vi "PH_BL-Master.PC _getVacLimits.vi"(0 "i ref in":refnum<vi>, 2 "Channelname":string="N/A", 3 "Value":dbl, 4 "no link":bool, 5 "error in (no error)":errorcluster) -> (14 "i ref out":refnum<vi>, 19 "error out":errorcluster)   [LabVIEW 2014, in "PH_BL-Master.lvlib"]
doc: "This VI writes the incoming information to own attributes."
uses:
  PH_BL-Master.lvlib
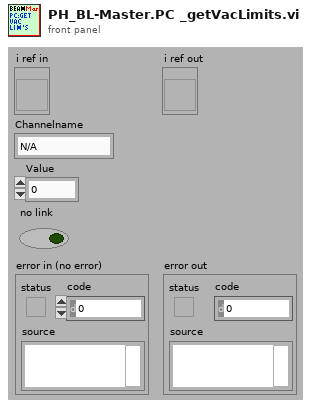
[diagram p1: front panel]
types:
  T1 = typedef "PH_BL-Master.lvlib/PH_BL-Master.i attribute.ctl" = cluster{"Remote controlled":bool, "Boolean Condition Service Subscriber":refnum<vi>[], "Picture Condition Service Subscriber":refnum<vi>[], "R2S":cluster{"GUI Ref":refnum<vi>, "State":bool}, "Vacua":cluster{"GUI Ref":refnum<vi>, "Limit":dbl, "Curr Value":dbl, "in range":bool}[], "O2 Inspection":cluster{"GUI Ref":refnum<vi>, "Concentration":dbl, "State":T2}[], "Boolean Status Service Subscriber":cluster{"GUI Ref":refnum<vi>, "Status":T2, "no Link?":bool, "Status Subscriber Class":T3}[], "Picture Status Service Subscriber":cluster{"GUI Ref":refnum<vi>, "Status":T2, "no Link?":bool, "Status Subscriber Class":T3}[], "6P 4Q Service Subscriber":cluster{"GUI Ref":refnum<vi>, "Selector":T4, "no Link?":bool}[], "Index of latest 6P 4Q changing Instance":i32, "Index of latest Picture Status changing Instance":i32, "Index of latest Boolean Status changing Instance":i32, "Vision ID on same Node":string, "Start Phase over?":bool, "GUI Ref Delete":refnum<vi>}
  T2 = typedef "PH_StatusHandler.lvlib/PH_StatusHandler.Status.ctl" = i16
  T3 = typedef "PH_BL-Master.lvlib/PH_BL-Master.Status Subscriber Class.ctl" = enum16{"unknown", "Switch", "BB", "6P Switch", "Switch GUI", "Switch and 6P State", "Force Sensor"}
  T4 = typedef "PH_4_Pos_Selector.lvlib/PH_4_Pos_Selector.Position Selector.ctl" = u16
  T5 = cluster{"GUI Ref":refnum<vi>, "Limit":dbl, "Curr Value":dbl, "in range":bool}[]
  T6 = cluster{"GUI Ref":refnum<vi>, "Limit":dbl, "Curr Value":dbl, "in range":bool}
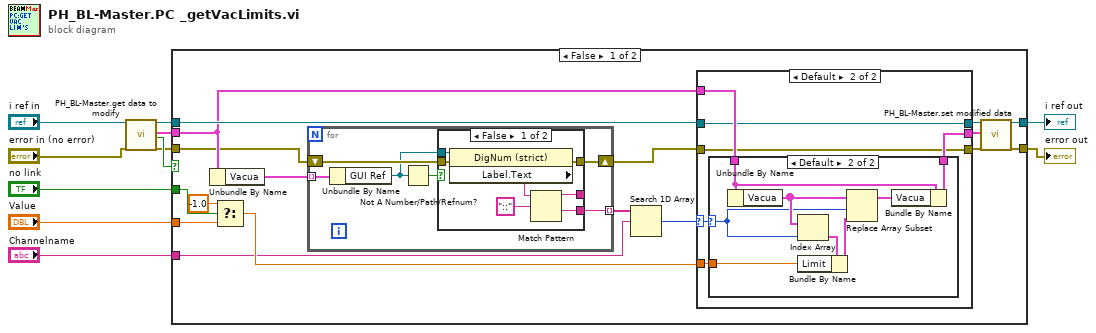
[diagram p0: block diagram]
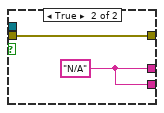
[diagram p4: hidden frame]
diagram:
  n1 = call "PH_BL-Master.get data to modify.vi"("i ref in"="i ref in", "error in (no error)"="error in (no error)") -> ("i ref out"=w6:refnum<vi>, "i attribute"=w10:T1, "timed out"=w11:bool, "error out"=w8:errorcluster)  [unwired: 14 in]
  n2 = case shown="False" w11 {
    tunnel: w6 -> [w22 w63]
    tunnel: [w28 w63] -> w7
    tunnel: w8 -> [w13 w62]
    tunnel: [w27 w62] -> w9
    tunnel: w10 -> [w15 _]
    tunnel: "Value" -> [w26 _]
    tunnel: "Channelname" -> [w12 _]
    tunnel: "no link" -> [w25 _]
    frame False {
      n3 = Unbundle By Name(w15) -> ("Vacua"=w20:T5)
      n4 = Select(t=-1.0, s=w25, f=w26) -> (s? t:f=w16:dbl)
      n5 = for {
        tunnel: w20 -> [w52] mode=indexing
        tunnel: [w51] -> w19 mode=indexing
        shift-right: [w50] -> w14
        shift-left: w13 -> [w49]
        n6 = Unbundle By Name(w52) -> ("GUI Ref"=w47:refnum<vi>)
        n7 = Not A Number/Path/Refnum?(number/path/refnum=w47) -> (NaN/Path/Refnum?=w48:bool)
        n8 = case shown="False" w48 {
          tunnel: w47 -> [w59 _]
          tunnel: [w56 w60] -> _
          tunnel: [w55 w60] -> w51
          tunnel: [w54 w61] -> w50
          tunnel: w49 -> [w53 w61]
          frame False {
            n9 = property class="DigNum (strict)"(reference=w59, error in=w53) -> (error out=w54:errorcluster, "Label.Text"=w58:string)  [unwired: 1 out]
            n10 = Match Pattern(string=w58, regular expression="::") -> (before substring=w56:string, after substring=w55:string)  [unwired: 1 in, 2 out]
          }
          frame True {
            w60 = "N/A" ("Label.Text")
          }
        }
      }
      n11 = Search 1D Array(1D array=w19, element=w12) -> (index of element=w17:i32)  [unwired: 1 in]
      n12 = case shown="Default" w17 {
        selector: w17 -> [_ w35]
        tunnel: w14 -> [w30 w33]
        tunnel: [w30 w33] -> w23
        tunnel: w22 -> [w31 w32]
        tunnel: [w31 w32] -> w21
        tunnel: [w29 w37] -> w18
        tunnel: w16 -> [_ w36]
        tunnel: w15 -> [w29 w34]
        frame -1 {
        }
        frame Default {
          n13 = case shown="Default" w35 {
            selector: w35 -> [_ w43]
            tunnel: [w38 w46] -> w37
            tunnel: w34 -> [w38 w39]
            tunnel: w36 -> [_ w40]
            frame -1 {
            }
            frame Default {
              n14 = Unbundle By Name(w39) -> ("Vacua"=w44:T5)
              n15 = Index Array(array=w44, index=w43) -> (element=w42:T6)
              n16 = Bundle By Name(cluster=w42, "Limit"=w40) -> (w41:T6)
              n17 = Replace Array Subset(array=w44, new element=w41, index=w43) -> (w45:T5)
              n18 = Bundle By Name(cluster=w39, "Vacua"=w45) -> (w46:T1)
            }
          }
        }
      }
      n19 = call "PH_BL-Master.set modified data.vi"("i ref in"=w21, "i attribute"=w18, "error in (no error)"=w23) -> ("i ref out"=w28:refnum<vi>, "error out"=w27:errorcluster)  [unwired: 15 in]
    }
    frame True {
    }
  }
  "error out" <- w9
  "i ref out" <- w7
